vi "GUID Lookup.vi"() -> ()   [LabVIEW 2016, in "LIN Frame Protection Addon Shared.lvlib"]
doc: "Use this Global VI to access the GUIDs assigned to the page resources of the Custom Device."
uses:
  LIN Frame Protection Addon Shared.lvlib
panel:
  in  "Protection Valid Channel Page Name":string="Valid"
  in  "Monitor Page Name":string="Monitor"
  in  "Generate Page Name":string="Generate"
  in  "Protection Valid Channel GUID":string="9276a97d-3f8a-408d-abe9-bee8bcaeaa49"
  in  "Monitor GUID":string="46c0c29d-91f6-4a25-a156-b8ef24eac378"
  in  "Generate GUID":string="f13b48ba-08da-41b2-b56f-dc3afba5b864"
  in  "Enable Disable GUID":string="4733d1e7-fc02-4e27-be4e-9d2e12f6fe6f"
  in  "Custom Device GUID_Disabled":string="ac3d5221-c9c0-44f4-a291-06920e8a9c9a"
  in  "Rolling Counter Value GUID":string="7762d13c-0e79-4a98-8860-3f1fdd9b969e"
  in  "Protection Value GUID":string="6cc69156-b54d-4826-9e4e-4b8a23c5091b"
  in  "Rolling Counter Value":string="Rolling Counter"
  in  "Protection Value":string="Protection"
  in  "Frame Configuration":string="Frame Configuration Settings"
  in  "Frame Configuration Page Name":string="Frame Configuration"
  in  "Frame Configuration GUID":string="080faed8-00b0-4df2-aec4-78e1bf3caf32"
  in  "Custom Device GUID":string="ce747db1-c753-4820-92b9-411d84571b92"
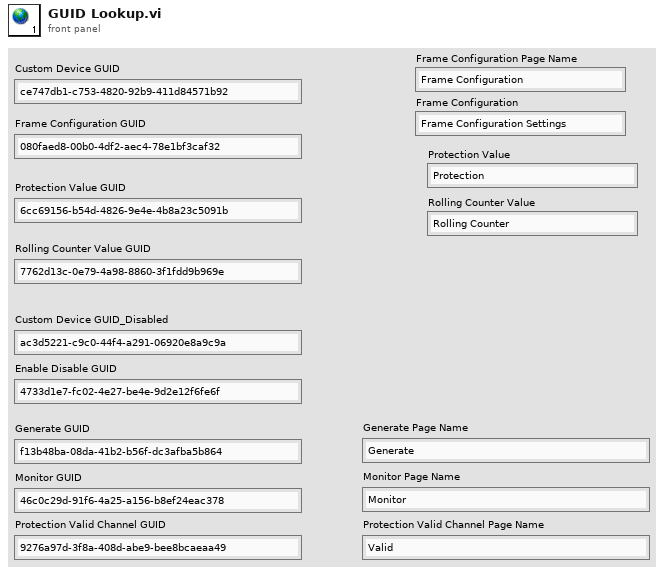
[diagram p1: front panel]
diagram:
